vi "Baratron.vi"() -> ()   [LabVIEW 2011]
panel:
  out "Boolean 24":bool
  out "Boolean 23":bool
  out "Boolean 22":bool
  out "Boolean 21":bool
  out "Boolean 20":bool
  out "Boolean 19":bool
  out "Boolean 18":bool
  out "Boolean 17":bool
  out "Boolean 16":bool
  out "Boolean 15":bool
  out "Boolean 14":bool
  out "Boolean 13":bool
  out "Boolean 12":bool
  out "Boolean 11":bool
  out "Boolean 10":bool
  out "Boolean 9":bool
  out "Boolean 8":bool
  out "Boolean 7":bool
  out "Boolean 6":bool
  out "Boolean 5":bool
  out "Boolean 4":bool
  out "Boolean 3":bool
  out "Boolean 2":bool
  out "Boolean":bool
  out "Baratron 92\n(%)":dbl
  out "Baratron 91\n(%)":dbl
  out "Baratron 90\n(%)":dbl
  out "Baratron 92\n(Counts)":i16
  out "Baratron 91\n(Counts)":i16
  out "Baratron 90\n(Counts)":i16
  in  "Full Scale":i16=23405
  in  "Stop Button":bool
  in  "BAR92 Byte 2":u8
  in  "BAR92 Byte 1":u8
  in  "BAR92 Byte 0":u8
  in  "BAR91 Byte 2":u8
  in  "BAR91 Byte 1":u8
  in  "BAR91 Byte 0":u8
  in  "BAR90 Byte 2":u8
  in  "BAR90 Byte 1":u8
  in  "BAR90 Byte 0":u8
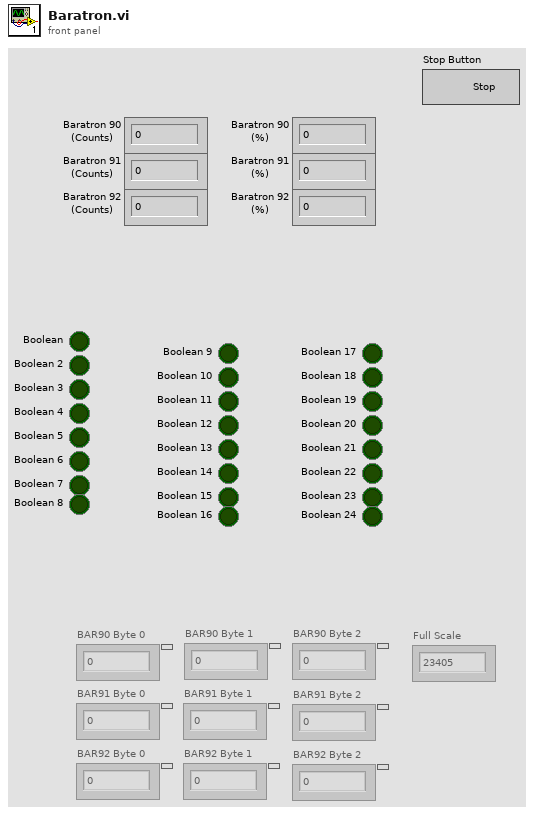
[diagram p1: front panel]
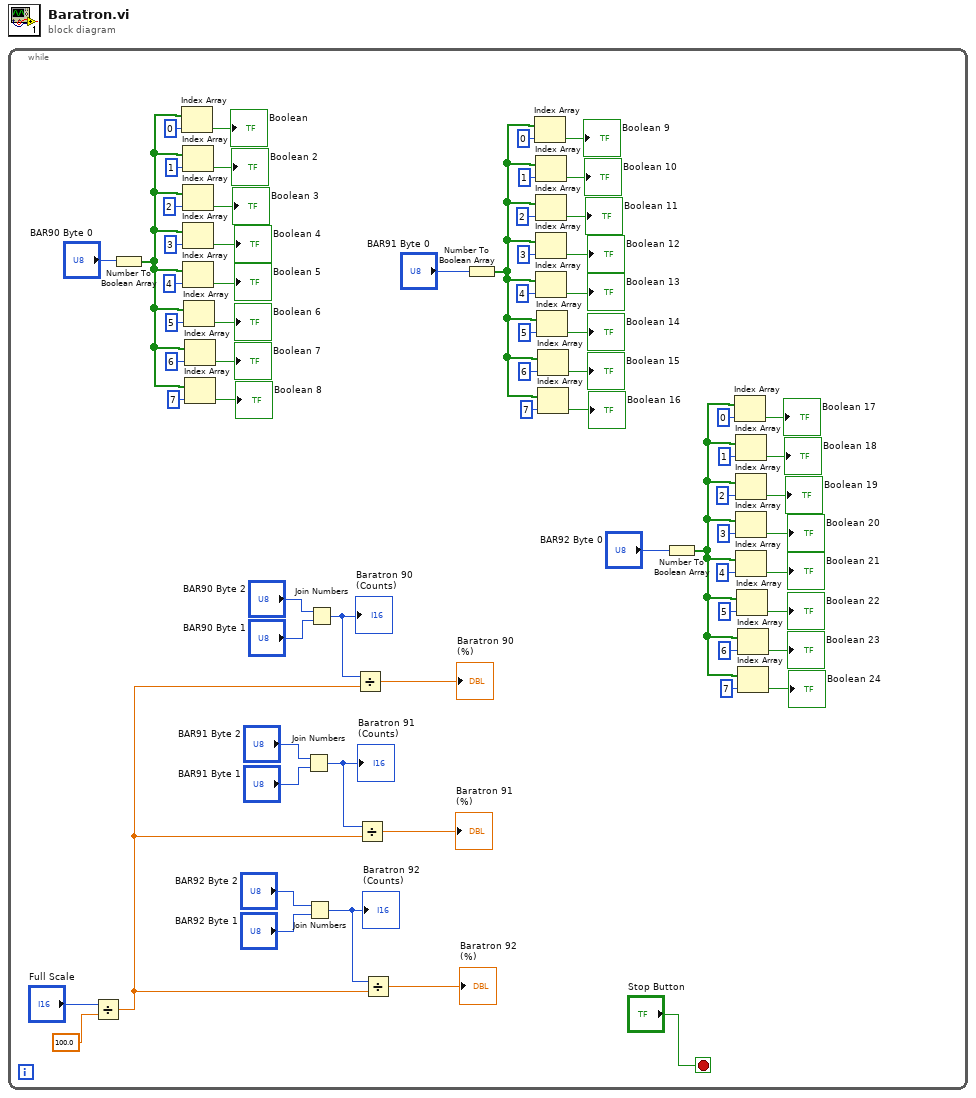
[diagram p0: block diagram]
diagram:
  n1 = while {
    stop <- "Stop Button" stop-if-true
    n2 = Divide(x="Full Scale", y=100.0) -> (x/y=w55:dbl)
    n3 = Number To Boolean Array(number="BAR90 Byte 0") -> (Boolean array=w37:bool[])
    n4 = Index Array(array=w37, index=0) -> (element=→"Boolean":bool)
    n5 = Index Array(array=w37, index=1) -> (element=→"Boolean 2":bool)
    n6 = Index Array(array=w37, index=2) -> (element=→"Boolean 3":bool)
    n7 = Index Array(array=w37, index=3) -> (element=→"Boolean 4":bool)
    n8 = Index Array(array=w37, index=4) -> (element=→"Boolean 5":bool)
    n9 = Index Array(array=w37, index=5) -> (element=→"Boolean 6":bool)
    n10 = Index Array(array=w37, index=6) -> (element=→"Boolean 7":bool)
    n11 = Index Array(array=w37, index=7) -> (element=→"Boolean 8":bool)
    n12 = Join Numbers(hi="BAR91 Byte 2", lo="BAR91 Byte 1") -> ((hi.lo)=w62:u16)
    "Baratron 91\n(Counts)" <- w62
    n13 = Join Numbers(hi="BAR92 Byte 2", lo="BAR92 Byte 1") -> ((hi.lo)=w61:u16)
    "Baratron 92\n(Counts)" <- w61
    n14 = Join Numbers(hi="BAR90 Byte 2", lo="BAR90 Byte 1") -> ((hi.lo)=w63:u16)
    "Baratron 90\n(Counts)" <- w63
    n15 = Divide(x=w63, y=w55) -> (x/y=→"Baratron 90\n(%)":dbl)
    n16 = Divide(x=w62, y=w55) -> (x/y=→"Baratron 91\n(%)":dbl)
    n17 = Divide(x=w61, y=w55) -> (x/y=→"Baratron 92\n(%)":dbl)
    n18 = Number To Boolean Array(number="BAR91 Byte 0") -> (Boolean array=w20:bool[])
    n19 = Index Array(array=w20, index=0) -> (element=→"Boolean 9":bool)
    n20 = Index Array(array=w20, index=1) -> (element=→"Boolean 10":bool)
    n21 = Index Array(array=w20, index=2) -> (element=→"Boolean 11":bool)
    n22 = Index Array(array=w20, index=3) -> (element=→"Boolean 12":bool)
    n23 = Index Array(array=w20, index=4) -> (element=→"Boolean 13":bool)
    n24 = Index Array(array=w20, index=5) -> (element=→"Boolean 14":bool)
    n25 = Index Array(array=w20, index=6) -> (element=→"Boolean 15":bool)
    n26 = Index Array(array=w20, index=7) -> (element=→"Boolean 16":bool)
    n27 = Number To Boolean Array(number="BAR92 Byte 0") -> (Boolean array=w2:bool[])
    n28 = Index Array(array=w2, index=0) -> (element=→"Boolean 17":bool)
    n29 = Index Array(array=w2, index=1) -> (element=→"Boolean 18":bool)
    n30 = Index Array(array=w2, index=2) -> (element=→"Boolean 19":bool)
    n31 = Index Array(array=w2, index=3) -> (element=→"Boolean 20":bool)
    n32 = Index Array(array=w2, index=4) -> (element=→"Boolean 21":bool)
    n33 = Index Array(array=w2, index=5) -> (element=→"Boolean 22":bool)
    n34 = Index Array(array=w2, index=6) -> (element=→"Boolean 23":bool)
    n35 = Index Array(array=w2, index=7) -> (element=→"Boolean 24":bool)
  }
